vi "ArrDataWriteTxt.vi"(0 "DataFileRef":refnum<file>, 9 "NewDataIn":dbl[][](array[numeric]) format="%#_16g", 11 "error in (no error)":errorcluster) -> (4 "DataFileRef Out":refnum<file>, 10 "NewDataOut":dbl[][](array[numeric]) format="%#_16g", 15 "error out":errorcluster)   [LabVIEW 2019]
doc: "Ce VI sauvegarde les données d'acquisition pour en garder une copie de sécurité qui peut être rappeller en cas de panne."
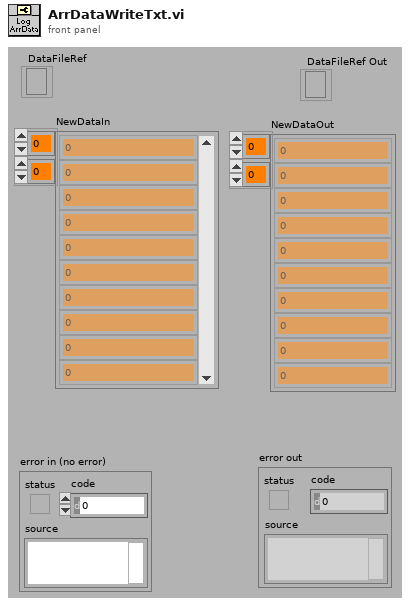
[diagram p1: front panel]
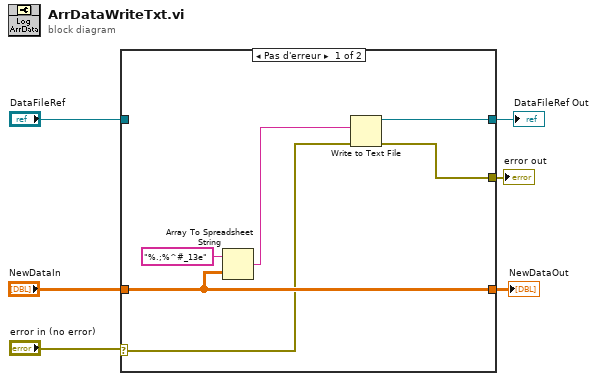
[diagram p0: block diagram]
diagram:
  n1 = case shown="Pas d'erreur" "error in (no error)" {
    selector: "error in (no error)" -> [w9 w15]
    tunnel: "NewDataIn" -> [w12 w14]
    tunnel: [w10 w15] -> w4
    tunnel: [w12 w14] -> w3
    tunnel: "DataFileRef" -> [_ w13]
    tunnel: [w8 w13] -> w1
    frame No Error {
      n2 = Array To Spreadsheet String(array=w12, 3:"%.;%^#_13e" ("chaîne de format")) -> (spreadsheet string=w7:string)  [unwired: 1 in]
      n3 = Write to Text File(text=w7, error in=w9) -> (refnum out=w8:refnum<file>, error out=w10:errorcluster)  [unwired: 2 in, 1 out]
    }
    frame Error {
    }
  }
  "NewDataOut" <- w3
  "error out" <- w4
  "DataFileRef Out" <- w1
